vi "FB Switch Output No Term No Var.vi"(8 "error in":errorcluster) -> (0 "error out":errorcluster)   [LabVIEW 2017]
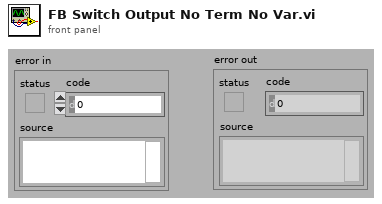
[diagram p1: front panel]
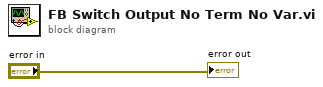
[diagram p0: block diagram]
diagram:
  "error out" <- "error in"
